vi "Sort Groups by Priority.vi"(8 "error in (no error)":errorcluster, 11 "Scheduler Plugin Bundle in":refnum<class "Scheduler Plugin Bundle.lvclass">) -> (0 "error out":errorcluster, 3 "Scheduler Plugin Bundle out":refnum<class "Scheduler Plugin Bundle.lvclass">)   [LabVIEW 2017, in "DSF Core.lvlib" / "Scheduler Plugin Bundle.lvclass"]
uses:
  Scheduler Plugin Bundle.lvclass
  Scheduler Plugin Bundle.lvclass/Scheduler Plugin Bundle.ctl
  Scheduler Transfer Group Bundle.lvclass
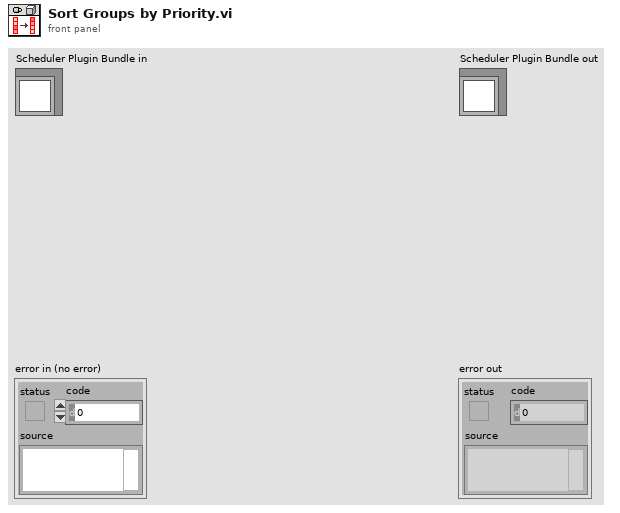
[diagram p1: front panel]
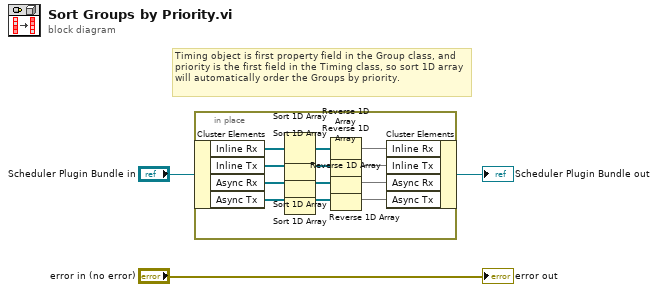
[diagram p0: block diagram]
diagram:
  # "Timing object is first property field in the Group class, and priority is the first field in the Timing class, so sort 1D array will automatically order the Groups by priority."
  n1 = in-place {
    n2 = in-place-cluster #1("Scheduler Plugin Bundle in") -> ("Inline Rx"=w15:refnum<class "Scheduler Transfer Group Bundle.lvclass">[], "Inline Tx"=w9:refnum<class "Scheduler Transfer Group Bundle.lvclass">[], "Async Rx"=w8:refnum<class "Scheduler Transfer Group Bundle.lvclass">[], "Async Tx"=w7:refnum<class "Scheduler Transfer Group Bundle.lvclass">[])
    n3 = Sort 1D Array(array=w15) -> (sorted array=w14:refnum<class "Scheduler Transfer Group Bundle.lvclass">[])
    n4 = Sort 1D Array(array=w9) -> (sorted array=w10:refnum<class "Scheduler Transfer Group Bundle.lvclass">[])
    n5 = Sort 1D Array(array=w8) -> (sorted array=w12:refnum<class "Scheduler Transfer Group Bundle.lvclass">[])
    n6 = Sort 1D Array(array=w7) -> (sorted array=w11:refnum<class "Scheduler Transfer Group Bundle.lvclass">[])
    n7 = Reverse 1D Array(array=w14) -> (reversed array=w13:refnum<class "Scheduler Transfer Group Bundle.lvclass">[])
    n8 = Reverse 1D Array(array=w10) -> (reversed array=w4:refnum<class "Scheduler Transfer Group Bundle.lvclass">[])
    n9 = Reverse 1D Array(array=w12) -> (reversed array=w5:refnum<class "Scheduler Transfer Group Bundle.lvclass">[])
    n10 = Reverse 1D Array(array=w11) -> (reversed array=w6:refnum<class "Scheduler Transfer Group Bundle.lvclass">[])
    n11 = in-place-cluster #1("Inline Rx"=w13, "Inline Tx"=w4, "Async Rx"=w5, "Async Tx"=w6) -> (→"Scheduler Plugin Bundle out":refnum<class "Scheduler Plugin Bundle.lvclass">)
  }
  "error out" <- "error in (no error)"
